vi "unhandled message received.vi"(9 "unhandled message":string, 11 "RT Queues":T1) -> ()   [LabVIEW 2018]
uses:
  Type Defs/Queues cluster.ctl
  ICL-LabVIEW_General/Message Scheduler/message scheduler.lvclass
  Queue VIs/En-queue RT comms element.vi
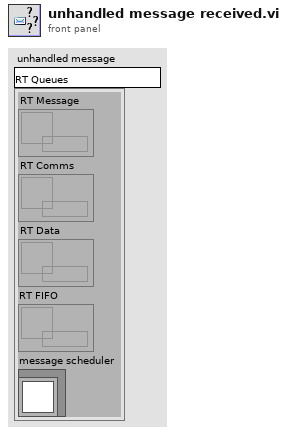
[diagram p1: front panel]
types:
  T1 = typedef "Queues cluster.ctl" = cluster{"RT Message":refnum<queue>, "RT Comms":refnum<queue>, "RT Data":refnum<queue>, "RT FIFO":refnum<queue>, "message scheduler":refnum<class "message scheduler.lvclass">}
  T2 = cluster{"seconds since 1Jan1904":timestamp, "type":string, "Variant":variant}
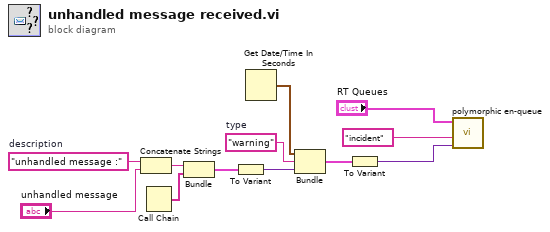
[diagram p0: block diagram]
diagram:
  w6 = "warning"  # type
  w9 = "unhandled message :"  # description
  n1 = Concatenate Strings(w9, "unhandled message") -> (w10:string)
  n2 = Call Chain() -> (call chain=w12:string[])
  n3 = Bundle(w10, "call chain"=w12) -> (w5:cluster{string, "call chain":string[]})  [unwired: 1 in]
  n4 = To Variant(anything=w5) -> (Variant=w4:variant)
  n5 = Get Date/Time In Seconds() -> (seconds since 1Jan1904=w1:timestamp)
  n6 = Bundle("seconds since 1Jan1904"=w1, "type"=w6, "Variant"=w4) -> (w3:T2)  [unwired: 1 in]
  n7 = To Variant(anything=w3) -> (Variant=w2:variant)
  n8 = call-poly "polymorphic en-queue.vi"("Data"=w2, "Message"="incident", "RT Queues"="RT Queues") -> ()  [unwired: 8 in, 1 out]
